vi "Stop Core.vi"(10 "final error code":i32, 11 "LeakyViewable in":refnum<class "LeakyViewable.lvclass">) -> (3 "LeakyViewable out":refnum<class "LeakyViewable.lvclass">)   [LabVIEW 2017, in "LeakyViewable.lvlib" / "LeakyViewable.lvclass"]
doc: "(<B>Filename</B>: Actor Framework.lvlib:Actor.lvclass:Stop Core.vi)\n\nDefines what the actor does before it stops. Use the <B>final error code</B> input to determine whether the actor shut down in response to an error.\n\nBy default, this method does nothing. A descendant class may override it to define behavior, such as shutting down any processes the actor initiated in its override of the Actor Core method.\n\n<License>\nCopyright © 2017 Composed Systems, LLC | All rights reserved\nwww.composed.io\n\nAuthor: Ethan Stern <ethan.stern@composed.io>\n\nThis software is provided \"AS IS\" WITHOUT WARRANTIES, either express or implied, AND IS FOR EDUCATIONAL PURPOSES ONLY.\n</License>"
uses:
  LeakyViewable.lvclass
  Leak Location.ctl
  Source/IViewable/IViewable/IViewable.lvclass
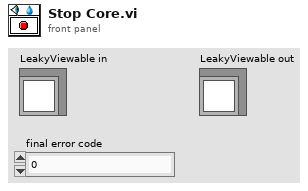
[diagram p1: front panel]
types:
  T1 = typedef "LeakyViewable.lvlib/LeakyViewable.lvclass/Leak Location.ctl" = enum16{"Pre Launch Init", "Entering Actor Core", "Actor Core", "Exiting Actor Core", "Stop Core", "Handle Error"}
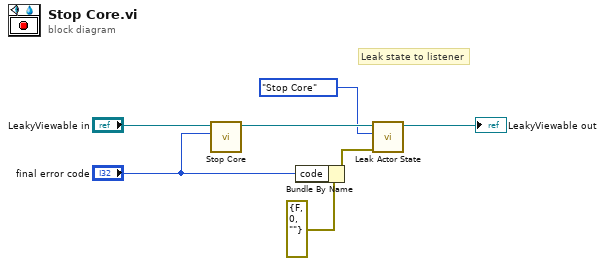
[diagram p0: block diagram]
diagram:
  # "Leak state to listener"
  n1 = call-parent "Stop Core.vi"("final error code"="final error code", "IViewable in"="LeakyViewable in") -> ("IViewable out"=w7:refnum<class "LeakyViewable.lvclass">)  [unwired: 9 in]
  n2 = Bundle By Name(cluster=errorcluster {"status"=FALSE, "code"=0, "source"=""} ("error in (no error)"), "code"="final error code") -> (w3:errorcluster)
  n3 = call "Leak Actor State.vi"("error in (no error)"=w3, "Location"=Leak_Location."Stop Core", "ViewableOne in"=w7) -> ("ViewableOne out"=→"LeakyViewable out":refnum<class "LeakyViewable.lvclass">)  [unwired: 7 in, 1 out]
